vi "Write U16.vi"(10 "U16":u16, 11 "Event in":refnum<class "Event U16.lvclass">) -> (3 "Event out":refnum<class "Event U16.lvclass">)   [LabVIEW 2016, in "Event Source.lvlib" / "Event U16.lvclass"]
uses:
  Event U16.lvclass
  Event U16.lvclass/Event U16.ctl
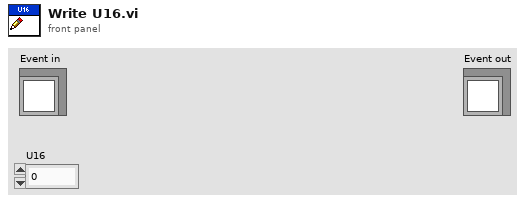
[diagram p1: front panel]
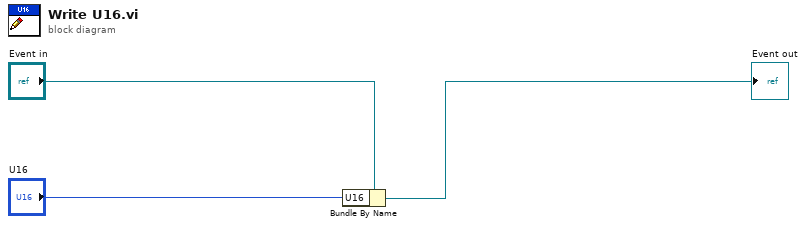
[diagram p0: block diagram]
diagram:
  n1 = Bundle By Name(cluster="Event in", "U16"="U16") -> (→"Event out":refnum<class "Event U16.lvclass">)
